vi "LWXPS_PositionerMotionDoneSet.vi"(0 "Positioner Name":string, 1 "Position window":dbl, 2 "Velocity window":dbl, 3 "Checking time":dbl, 4 "Mean period":dbl, 5 "Motion done time out":dbl, 6 "XPS Reference IN":refnum<k24>, 7 "LabVIEW error IN":errorcluster) -> (14 "XPS Reference OUT":refnum<k24>, 15 "Returned error code":i32, 18 "XPS Error String":string, 19 "LabVIEW error OUT":errorcluster)   [LabVIEW 2014]
uses:
  D:/XPSQ8_LabView_Library/Development/Source/Dll/Newport.XPS.CommandInterface.dll
  Dll/Newport.XPS.CommandInterface.dll
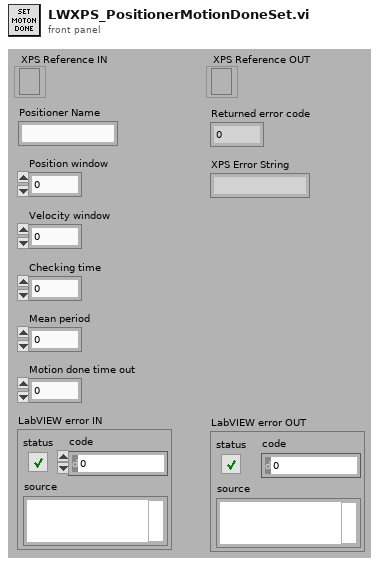
[diagram p1: front panel]
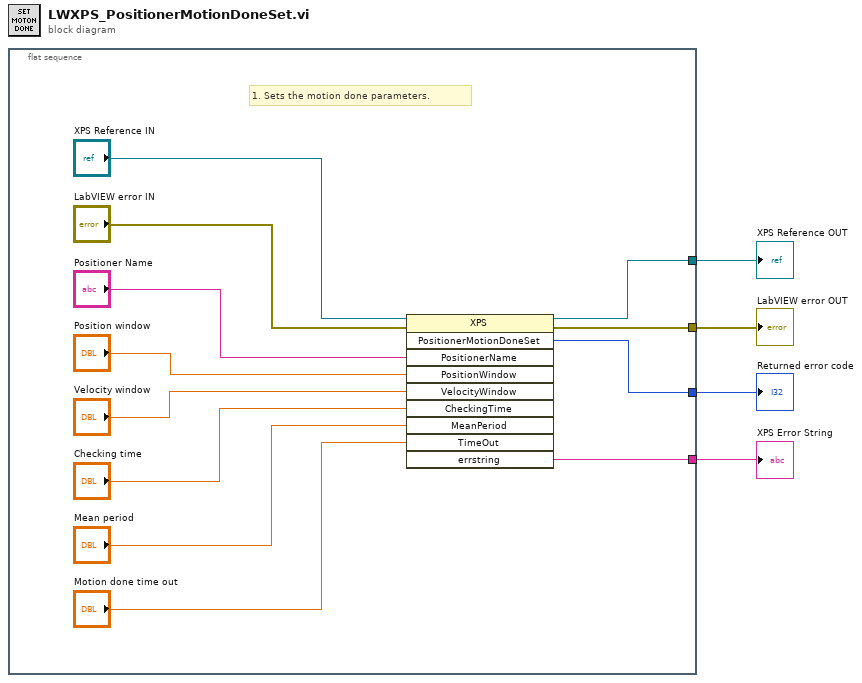
[diagram p0: block diagram]
diagram:
  n1 = flat-sequence {
    tunnel: [w12] -> w4
    tunnel: [w15] -> w3
    tunnel: [w14] -> w2
    tunnel: [w11] -> w1
    frame #0 {
      # "1. Sets the motion done parameters."
      n2 = invoke class="XPS" method="PositionerMotionDoneSet"(reference="XPS Reference IN", error in="LabVIEW error IN", "PositionerName"="Positioner Name", "PositionWindow"="Position window", "VelocityWindow"="Velocity window", "CheckingTime"="Checking time", "MeanPeriod"="Mean period", "TimeOut"="Motion done time out") -> (reference out=w12:refnum<k24>, error out=w15:errorcluster, "PositionerMotionDoneSet"=w14:i32, "errstring"=w11:string)  [unwired: 2 in, 6 out]
    }
  }
  "XPS Error String" <- w1
  "XPS Reference OUT" <- w4
  "LabVIEW error OUT" <- w3
  "Returned error code" <- w2
